vi "EOL Initialize Power Supplies.vi"(7 "Volt Limit":dbl=13.5, 8 "Error In":errorcluster, 9 "power supply model":T1, 10 "No. of Power Supplies":i32=1, 11 "VISA resource name":refnum<visa-resource-name>) -> (0 "error out":errorcluster)   [LabVIEW 2018]
doc: "This VI Initializes all 12 of the lambda Power Supplies"
uses:
  power supply types.ctl
  04.SubVI's/Fergus/ZUP_Current/Def Ctrl/CMD Type.ctl
  Instance           1 37Saved   Initialize All Power Supplies .vi
  ITECH/IT-M3100.lvlib
panel:
  out ".not. x?":bool
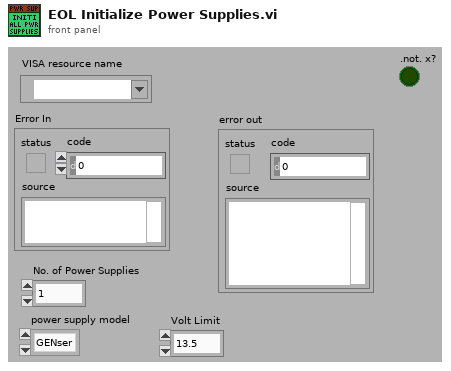
[diagram p1: front panel]
types:
  T1 = typedef "power supply types.ctl" = enum16{"GENser", "ZUPser", "GENeth", "Manual", "ITECH"}
  T2 = cluster{"Baud Rate":u32, "Parity":u16, "Data Bits":u16, "Stop Bits":u16}
  T3 = typedef "CMD Type.ctl" = enum16{"Default", "SetADR", "SetRMT", "SetVOL", "SetCUR", "SetOUT", "CheckREV", "CheckRMT", "CheckVOL", "CkeckCUR", "CheckOUT"}
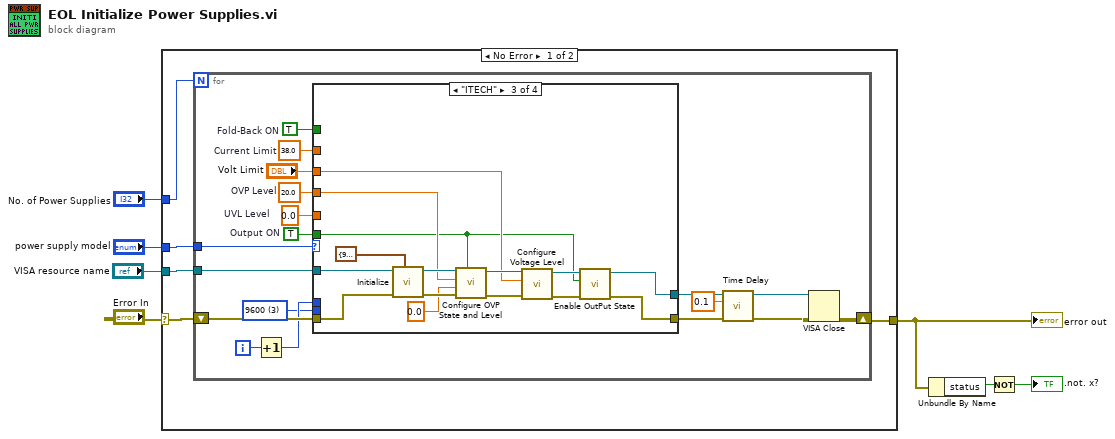
[diagram p0: block diagram]
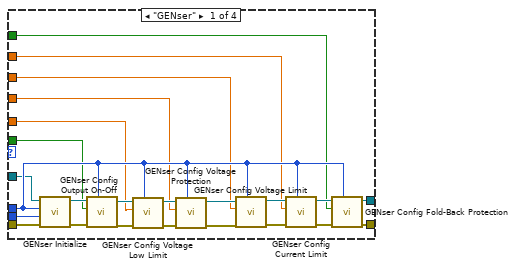
[diagram p2: hidden frame]
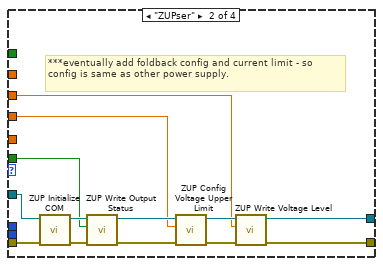
[diagram p3: hidden frame]
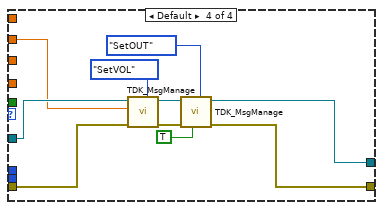
[diagram p4: hidden frame]
diagram:
  n1 = case shown="No Error" "Error In" {
    selector: "Error In" -> [w11 w92]
    tunnel: [w12 w92] -> w5
    tunnel: "VISA resource name" -> [w8 _]
    tunnel: "No. of Power Supplies" -> [w10 _]
    tunnel: "power supply model" -> [w9 _]
    frame No Error {
      n2 = for {
        N: w10 -> [_]
        shift-right: [w15] -> w12
        shift-left: w11 -> [w29]
        tunnel: w9 -> [w23]
        tunnel: w8 -> [w14]
        i -> [w28]
        w18 = TRUE  # Output ON
        w19 = TRUE  # Fold-Back ON
        w20 = 38.0  # Current Limit
        w21 = 20.0  # OVP Level
        w22 = 0.0  # UVL Level
        w24 = u16 3 items=["1200", "2400", "4800", "9600", "19200"] ("BAUD")
        n3 = Increment(x=w28) -> (x+1=w27:i32)
        n4 = case shown="\"ITECH\"" w23 {
          tunnel: w29 -> [w53 w66 w77 w84]
          tunnel: w27 -> [w40 _ _ _]
          tunnel: [w39 w55 w68 w82] -> w26
          tunnel: [w38 w56 w69 w83] -> w17
          tunnel: w24 -> [w37 _ _ _]
          tunnel: w22 -> [w36 _ _ _]
          tunnel: w21 -> [w35 w60 w76 _]
          tunnel: "Volt Limit" -> [w34 w57 w72 w85]
          tunnel: w20 -> [w33 _ _ _]
          tunnel: w19 -> [w32 _ _ _]
          tunnel: w18 -> [w31 w63 w67 _]
          tunnel: w14 -> [w30 w54 w81 w86]
          frame "GENser" {
            n5 = call "GENser Initialize.vi"("error in (no error)"=w53, "BAUD"=w37, "GEN Addr"=w40, "VISA resource name"=w30) -> ("error out"=w52:errorcluster, "VISA out"=w51:refnum<visa-resource-name>)  [unwired: 6 in]
            n6 = call "GENser Config Output On-Off.vi"("GEN Addr"=w40, "error"=w52, "Output ON"=w31, "VISA"=w51) -> ("error out"=w48:errorcluster, "VISA out"=w47:refnum<visa-resource-name>)  [unwired: 6 in]
            n7 = call "GENser Config Voltage Low Limit.vi"("GEN Addr"=w40, "error"=w48, "UVL Level"=w36, "VISA"=w47) -> ("error out"=w50:errorcluster, "VISA out"=w49:refnum<visa-resource-name>)  [unwired: 6 in]
            n8 = call "GENser Config Voltage Protection.vi"("GEN Addr"=w40, "error"=w50, "OVP Level"=w35, "VISA"=w49) -> ("error out"=w46:errorcluster, "VISA out"=w45:refnum<visa-resource-name>)  [unwired: 6 in]
            n9 = call "GENser Config Voltage Limit.vi"("GEN Addr"=w40, "error"=w46, "Volt Limit"=w34, "VISA"=w45) -> ("error out"=w44:errorcluster, "VISA out"=w43:refnum<visa-resource-name>)  [unwired: 6 in]
            n10 = call "GENser Config Current Limit.vi"("GEN Addr"=w40, "error"=w44, "Current Limit"=w33, "VISA"=w43) -> ("error out"=w42:errorcluster, "VISA out"=w41:refnum<visa-resource-name>)  [unwired: 6 in]
            n11 = call "GENser Config Fold-Back Protection.vi"("GEN Addr"=w40, "error"=w42, "Fold-Back ON"=w32, "VISA"=w41) -> ("error out"=w39:errorcluster, "VISA out"=w38:refnum<visa-resource-name>)  [unwired: 6 in]
          }
          frame "ZUPser" {
            # "***eventually add foldback config and current limit - so config is same as other power supply."
            n12 = call "ZUP Initialize COM.vi"("error in (no error)"=w66, "VISA resource name"=w54) -> ("error out"=w64:errorcluster, "VISA OUT"=w65:refnum<visa-resource-name>)  [unwired: 8 in]
            n13 = call "ZUP Write Output Status.vi"("error in (no error)"=w64, "ON/OFF"=w63, "VISA resource name"=w65) -> ("error out"=w61:errorcluster, "VISA OUT"=w62:refnum<visa-resource-name>)  [unwired: 6 in, 1 out]
            n14 = call "ZUP Config Voltage Upper Limit.vi"("error in (no error)"=w61, "Voltage Limit"=w60, "VISA resource name"=w62) -> ("error out"=w58:errorcluster, "VISA OUT"=w59:refnum<visa-resource-name>)  [unwired: 6 in, 1 out]
            n15 = call "ZUP Write Voltage Level.vi"("error in (no error)"=w58, "Voltage"=w57, "VISA resource name"=w59) -> ("error out"=w55:errorcluster, "VISA OUT"=w56:refnum<visa-resource-name>)  [unwired: 6 in, 1 out]
          }
          frame "ITECH" {
            n16 = call "Initialize.vi"("Serial Configuration"=T2 {"Baud Rate"=9600, "Parity"=0, "Data Bits"=8, "Stop Bits"=10}, "error in"=w77, "VISA resource name"=w81) -> ("error out"=w78:errorcluster, "VISA resource name out"=w79:refnum<visa-resource-name>)  [unwired: 7 in]
            n17 = call "Configure OVP State and Level.vi"("State"=w67, "error in"=w78, "OVP Delay(S)"=0.0, "OVP Level(V)"=w76, "VISA resource name"=w79) -> ("error out"=w73:errorcluster, "VISA resource name out"=w74:refnum<visa-resource-name>)  [unwired: 5 in]
            n18 = call "Configure Voltage Level.vi"("error in"=w73, "Level(V)"=w72, "VISA resource name"=w74) -> ("error out"=w70:errorcluster, "VISA resource name out"=w71:refnum<visa-resource-name>)  [unwired: 7 in]
            n19 = call "Enable OutPut State.vi"("error in"=w70, "State"=w67, "VISA resource name"=w71) -> ("error out"=w68:errorcluster, "VISA resource name out"=w69:refnum<visa-resource-name>)  [unwired: 7 in]
          }
          frame Default {
            n20 = call "TDK_MsgManage.vi"("CMD Type"=CMD_Type."SetVOL", "error in (no error)"=w84, "Voltage"=w85, "VISA resource name"=w86) -> ("error out"=w90:errorcluster, "VISA resource name"=w89:refnum<visa-resource-name>)  [unwired: 4 in, 2 out]
            n21 = call "TDK_MsgManage.vi"("CMD Type"=CMD_Type."SetOUT", "OUT?"=TRUE, "error in (no error)"=w90, "VISA resource name"=w89) -> ("error out"=w82:errorcluster, "VISA resource name"=w83:refnum<visa-resource-name>)  [unwired: 4 in, 2 out]
          }
        }
        n22 = call "Time Delay"("error in (no error)"=w26, "Delay Time (s)"=0.1) -> ("error out"=w16:errorcluster)  [unwired: 9 in]
        n23 = VISA Close(VISA resource name=w17, error in (no error)=w16) -> (error out=w15:errorcluster)
      }
    }
    frame Error {
    }
  }
  "error out" <- w5
  n24 = Unbundle By Name(w5) -> ("status"=w4:bool)
  n25 = Not(x=w4) -> (.not. x?=→".not. x?":bool)
